vi "Resolve Names Test.vi"() -> (2 "Pass?":bool)   [LabVIEW 2015, in "SystemLink Tag Module tests.lvlib"]
uses:
  SystemLink Tag Module tests.lvlib
  module/configuration/SystemLink configuration.lvclass
  module/configuration/SystemLink configuration.lvclass/SystemLink configuration.ctl
  module/configuration/Write Prepend Minion ID.vi
  module/execution/SystemLink runtime.lvclass
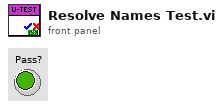
[diagram p1: front panel]
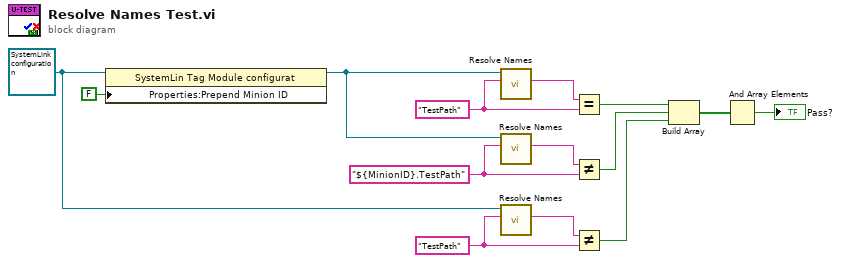
[diagram p0: block diagram]
diagram:
  w6 = "${MinionID}.TestPath" ("Path In")
  w12 = "TestPath" ("Path In")
  w13 = "TestPath" ("Path In")
  w3 = refnum<class "SystemLink configuration.lvclass"> refnum ("SystemLin Tag Module configuration")
  n1 = property class="SystemLin Tag Module configurat"(reference=w3, "Properties:Prepend Minion ID"=FALSE ("Prepend Minion ID")) -> (reference out=w2:refnum<class "SystemLink configuration.lvclass">)  [unwired: 1 in, 1 out]
  n2 = call "Resolve Names.vi"("Path In"=w13, "SystemLin Tag Module configuration"=w2) -> ("Path Out"=w14:string)  [unwired: 6 in, 1 out]
  n3 = call "Resolve Names.vi"("Path In"=w6, "SystemLin Tag Module configuration"=w2) -> ("Path Out"=w7:string)  [unwired: 6 in, 1 out]
  n4 = call "Resolve Names.vi"("Path In"=w12, "SystemLin Tag Module configuration"=w3) -> ("Path Out"=w11:string)  [unwired: 6 in, 1 out]
  n5 = Equal?(x=w14, y=w13) -> (x = y?=w10:bool)
  n6 = Not Equal?(x=w7, y=w6) -> (x != y?=w5:bool)
  n7 = Not Equal?(x=w11, y=w12) -> (x != y?=w4:bool)
  n8 = Build Array(w10, w5, w4) -> (w9:bool[])
  n9 = And Array Elements(Boolean array=w9) -> (logical AND=→"Pass?":bool)
